vi "ET2604 - Write To Register Floating Point.vi"(7 "Unit Address (1)":u8=1, 8 "error in (no error)":errorcluster, 9 "Data (0)":sgl format="%.3f", 10 "Register Address (0)":u16, 11 "VISA session":refnum<visa-resource-name>) -> (0 "error out":errorcluster, 3 "dup VISA session":refnum<visa-resource-name>)   [LabVIEW 2017]
doc: "This VI writes the values to the specified registers of specified unit."
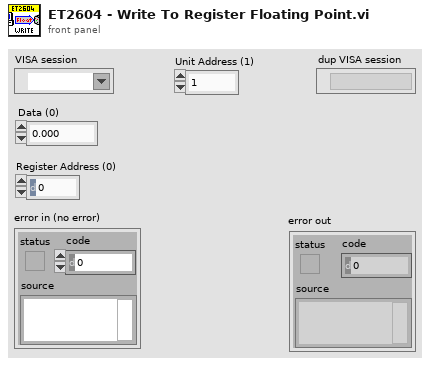
[diagram p1: front panel]
types:
  T1 = enum16{"By The Number of Bytes", "Copy Of the Sent Message"}
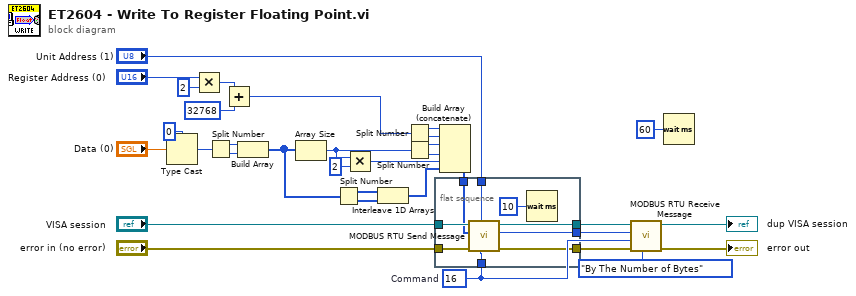
[diagram p0: block diagram]
diagram:
  w5 = u8 16  # Command
  n1 = Type Cast(type=0 ("y"), x="Data (0)") -> (*(type *) &x=w19:i32)
  n2 = Multiply(x="Register Address (0)", y=u16 2) -> (x*y=w14:u16)
  n3 = Split Number(x=w19) -> (hi(x)=w10:u16, lo(x)=w9:u16)
  n4 = Add(x=w14, y=u16 32768) -> (x+y=w11:u16)
  n5 = Build Array(w10, w9) -> (w16:u16[])
  n6 = Array Size(array=w16) -> (size(s)=w25:i32)
  n7 = Split Number(x=w16) -> (hi(x)=w21:u8[], lo(x)=w22:u8[])
  n8 = Multiply(x=w25, y=2) -> (x*y=w24:i32)
  n9 = Interleave 1D Arrays(w21, w22) -> (w20:u8[])
  n10 = Split Number(x=w11) -> (hi(x)=w30:u8, lo(x)=w29:u8)
  n11 = Split Number(x=w25) -> (hi(x)=w28:u16, lo(x)=w27:u16)
  n12 = flat-sequence {
    tunnel: "VISA session" -> [w39]
    tunnel: "error in (no error)" -> [w40]
    tunnel: [w36] -> w4
    tunnel: [w34] -> w7
    tunnel: w5 -> [w41]
    tunnel: w31 -> [w38]
    tunnel: [w35] -> w6
    tunnel: "Unit Address (1)" -> [w37]
    frame #0 {
      n13 = call "MODBUS RTU Send Message.vi"("Command (0)"=w41, "Unit Address (1)"=w37, "error in (no error)"=w40, "Message (empty array)"=w38, "VISA session"=w39) -> ("error out"=w36:errorcluster, "Length Of Sent MSG"=w35:u8, "dup VISA session"=w34:refnum<visa-resource-name>)  [unwired: 4 in]
      n14 = Wait (ms)(milliseconds to wait=u32 10) -> ()  [unwired: 1 out]
    }
  }
  n15 = Build Array (concatenate)(w30, w29, w28, w27, w24, w20) -> (w31:i32[])
  n16 = call "MODBUS RTU Receive Message.vi"("Receive Message Type (0: By The Number Of Bytes)"=T1."By The Number of Bytes" ("Receive Message Type"), "error in (no error)"=w4, "Sent Command (0)"=w5, "Length Of Sent MSG (0)"=w6, "VISA session"=w7) -> ("error out"=→"error out":errorcluster, "dup VISA session"=→"dup VISA session":refnum<visa-resource-name>)  [unwired: 4 in, 1 out]
  n17 = Wait (ms)(milliseconds to wait=u32 60) -> ()  [unwired: 1 out]
